vi "Fetch Multi Eval Meas List Segment SEM Margin Results.vi"(6 "Segment (1)":T2=1, 7 "Offset Frequency (Positive)":i32(ring)=1 items=["Negative", "Positive"], 8 "error in (no error)":errorcluster, 9 "Result Type (Current)":i32(ring) items=["Current"=0, "Average"=1, "Minimum"=5], 10 "Instance (1)":T3=1, 11 "VISA resource name":refnum<visa-resource-name>) -> (0 "error out":errorcluster, 1 "SEM Margin Results":cluster{"Margin X":dbl, "Margin Y":dbl}[](array[cluster]) {"Margin Y" format="%^.3e"; "Margin X" format="%^.3e"}, 2 "Reliability":T1, 3 "VISA resource name out":refnum<visa-resource-name>, 4 "Expired Statistics":i32, 5 "Out Of Tolerance":i32)   [LabVIEW 2020, in "Rohde&Schwarz CMWXP NR FR1 Measurement.lvlib"]
doc: "Return spectrum emission mask margin results for segment <no> in list mode. The results for the current, average and maximum traces (resulting in minimum margins) for negative and positive offset frequencies are available.\n\nAttributes:\nRSCMWXPNRFR1M_ATTR_FETCH_MULTI_EVAL_MEAS_LIST_SEGMENT_SEM_MARGIN_NEGATIVE_CURRENT_RESULTS\nRSCMWXPNRFR1M_ATTR_FETCH_MULTI_EVAL_MEAS_LIST_SEGMENT_SEM_MARGIN_NEGATIVE_AVERAGE_RESULTS\nRSCMWXPNRFR1M_ATTR_FETCH_MULTI_EVAL_MEAS_LIST_SEGMENT_SEM_MARGIN_NEGATIVE_MINIMUM_RESULTS\nRSCMWXPNRFR1M_ATTR_FETCH_MULTI_EVAL_MEAS_LIST_SEGMENT_SEM_MARGIN_POSITIVE_CURRENT_RESULTS\nRSCMWXPNRFR1M_ATTR_FETCH_MULTI_EVAL_MEAS_LIST_SEGMENT_SEM_MARGIN_POSITIVE_AVERAGE_RESULTS\nRSCMWXPNRFR1M_ATTR_FETCH_MULTI_EVAL_MEAS_LIST_SEGMENT_SEM_MARGIN_POSITIVE_MINIMUM_RESULTS\n\nRemote-control commands:\nFETCh:NRSub:MEAS<i>:MEValuation:LIST:SEGMent<no>:SEMask:MARGin:CURRent:NEGativ?\nFETCh:NRSub:MEAS<i>:MEValuation:LIST:SEGMent<no>:SEMask:MARGin:AVERage:NEGativ?\nFETCh:NRSub:MEAS<i>:MEValuation:LIST:SEGMent<no>:SEMask:MARGin:MINimum:NEGativ?\nFETCh:NRSub:MEAS<i>:MEValuation:LIST:SEGMent<no>:SEMask:MARGin:CURRent:POSitiv?\nFETCh:NRSub:MEAS<i>:MEValuation:LIST:SEGMent<no>:SEMask:MARGin:AVERage:POSitiv?\nFETCh:NRSub:MEAS<i>:MEValuation:LIST:SEGMent<no>:SEMask:MARGin:MINimum:POSitiv?"
uses:
  <instrlib>/Rohde&Schwarz CMWXP NR FR1 Measurement/Rohde&Schwarz CMWXP NR FR1 Measurement.lvlib
  <instrlib>/Rohde&Schwarz CMWXP NR FR1 Measurement/Private/_Instance.ctl
  <instrlib>/Rohde&Schwarz CMWXP NR FR1 Measurement/Private/_Segment.ctl
  <instrlib>/Rohde&Schwarz CMWXP NR FR1 Measurement/Private/_SegReliability.ctl
  <instrlib>/Rohde&Schwarz CMWXP NR FR1 Measurement/Private/rsidr_core.llb/rsidr_core.lvlib
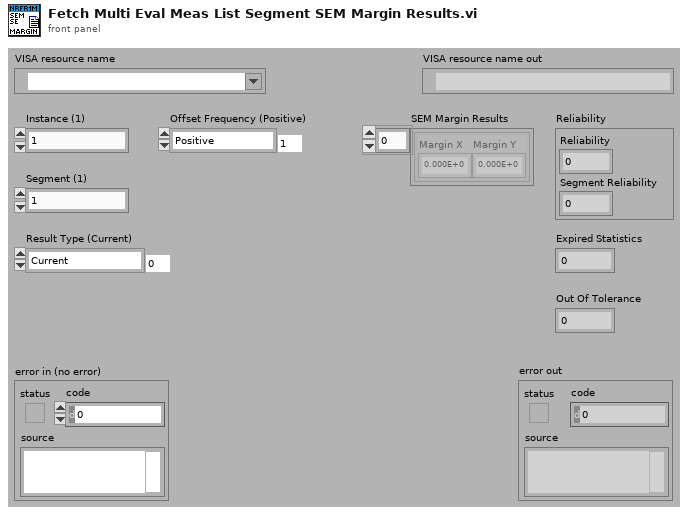
[diagram p1: front panel]
types:
  T1 = typedef "Rohde&Schwarz CMWXP NR FR1 Measurement.lvlib/_SegReliability.ctl" = cluster{"Reliability":i32, "Segment Reliability":i32}
  T2 = typedef "Rohde&Schwarz CMWXP NR FR1 Measurement.lvlib/_Segment.ctl" = i32
  T3 = typedef "Rohde&Schwarz CMWXP NR FR1 Measurement.lvlib/_Instance.ctl" = i32
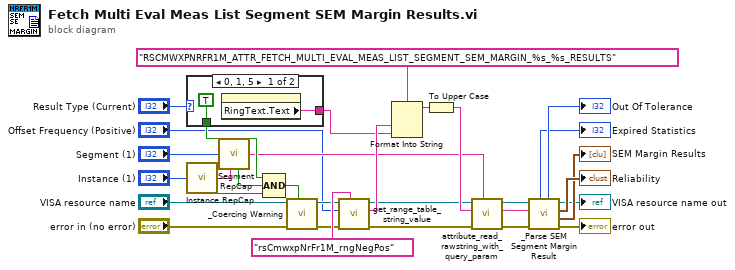
[diagram p0: block diagram]
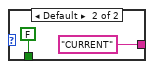
[diagram p2: hidden frame]
diagram:
  n1 = case shown="0, 1, 5" "Result Type (Current)" {
    tunnel: [w32 "CURRENT"] -> w20
    tunnel: [TRUE FALSE] -> w22
    frame 0, 1, 5 {
      n2 = property on="Result Type (Current)" class="Ring (strict)"() -> ("RingText.Text"=w32:string)  [unwired: 2 in, 2 out]
    }
    frame Default {
    }
  }
  n3 = call <instrlib>:"Instance RepCap.vi"("Instance In"="Instance (1)") -> ("In Range?"=w30:bool, "RepCap Identifier Out"=w29:string)  [unwired: 1 in]
  n4 = call <instrlib>:"Segment RepCap.vi"("Segment In"="Segment (1)", "RepCap String In (\"\")"=w29) -> ("In Range?"=w28:bool, "RepCap Identifier Out"=w18:string)
  n5 = Compound Arithmetic op=AND(w22, w28, w30) -> (w31:bool)
  n6 = call <instrlib>:"_Coercing Warning.vi"("In Range?"=w31, "error in (no error)"="error in (no error)", "VISA resource name"="VISA resource name") -> ("error out"=w25:errorcluster, "VISA resource name out"=w26:refnum<visa-resource-name>)  [unwired: 7 in]
  n7 = call <instrlib>:"get_range_table_string_value.vi"("Range Table ID in"="rsCmwxpNrFr1M_rngNegPos", "error in"=w25, "I32 input"="Offset Frequency (Positive)", "VISA resource name"=w26) -> ("error out"=w16:errorcluster, "String Value out"=w21:string, "VISA resource name out"=w17:refnum<visa-resource-name>)  [unwired: 5 in]
  n8 = Format Into String(format string="RSCMWXPNRFR1M_ATTR_FETCH_MULTI_EVAL_MEAS_LIST_SEGMENT_SEM_MARGIN_%s_%s_RESULTS", w21, w20) -> (resulting string=w23:string)  [unwired: 2 in, 1 out]
  n9 = To Upper Case(1:w23) -> (0:w19:string)
  n10 = call <instrlib>:"attribute_read_rawstring_with_query_param.vi"("Repeated Capability"=w18, "error in"=w16, "Attribute ID"=w19, "VISA resource name"=w17) -> ("error out"=w9:errorcluster, "Raw String out"=w8:string, "VISA resource name out"=w7:refnum<visa-resource-name>)  [unwired: 5 in]
  n11 = call <instrlib>:"_Parse SEM Segment Margin Result.vi"("error in (no error)"=w9, "Input String"=w8, "VISA resource name"=w7) -> ("error out"=→"error out":errorcluster, "SEM Margin Results"=→"SEM Margin Results":cluster{"Margin X":dbl, "Margin Y":dbl}[], "Reliability Results"=→"Reliability":T1, "VISA resource name out"=→"VISA resource name out":refnum<visa-resource-name>, "Out Of Tolerance"=→"Out Of Tolerance":i32, "Statistic Expired"=→"Expired Statistics":i32)  [unwired: 3 in]
